vi "loadDataNodeEnd.vi"(8 "error in (no error)":errorcluster, 10 "XML Refnum in":refnum<file>, 11 "FPGADMAChannelData in":refnum<class "FPGADMAChannelData.lvclass">) -> (0 "error out":errorcluster, 2 "XML Refnum out":refnum<file>, 3 "FPGADMAChannelData out":refnum<class "FPGADMAChannelData.lvclass">)   [LabVIEW 2013, in "FPGADMAChannelData.lvclass"]
doc: "Part of the file loading process. Occurs at the end of a node being loaded. Includes checking the end of the tag which has the format </tag>."
uses:
  FPGADMAChannelData.lvclass
  xCE/xceRootNode/xceRootNode.lvclass
  XML Parser/XML Parser.lvclass
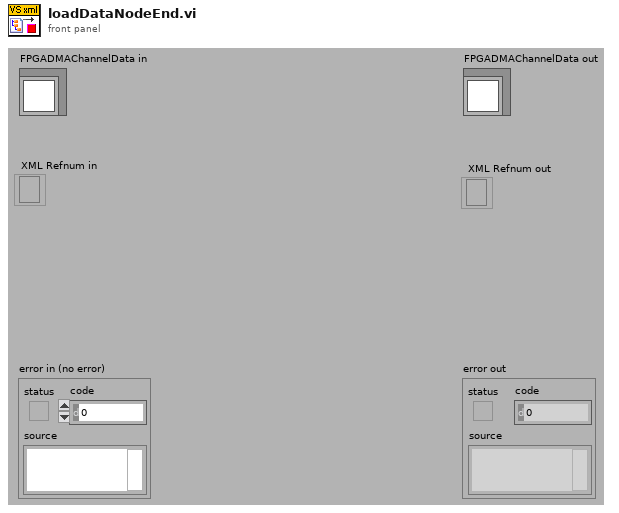
[diagram p1: front panel]
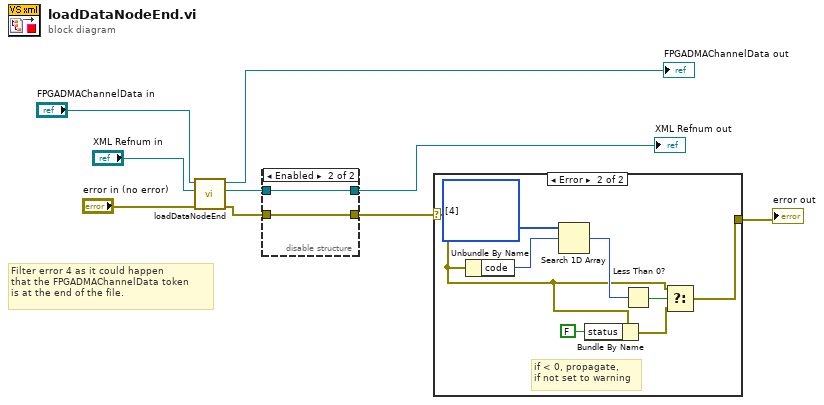
[diagram p0: block diagram]
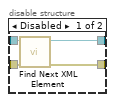
[diagram p2: hidden frame]
diagram:
  # "Filter error 4 as it could happen \nthat the FPGADMAChannelData token\nis at the end of the file."
  n1 = call-parent "loadDataNodeEnd.vi"("error in (no error)"="error in (no error)", "XML Refnum in"="XML Refnum in", "xceDataNode in"="FPGADMAChannelData in") -> ("error out"=w3:errorcluster, "XML Refnum out"=w4:refnum<file>, "xceDataNode out"=→"FPGADMAChannelData out":refnum<class "FPGADMAChannelData.lvclass">)  [unwired: 6 in]
  n2 = disable-structure shown="Enabled" {
    disable-tunnel: w4 -> [w13 w15]
    disable-tunnel: w3 -> [w12 w14]
    disable-tunnel: [w11 w15] -> w2
    disable-tunnel: [w10 w14] -> w1
    frame Disabled {
      n3 = call "Find Next XML Element.vi"("error in (no error)"=w12, "XML Fine In"=w13) -> ("error out"=w10:errorcluster, "XML Fine Out"=w11:refnum<file>)  [unwired: 7 in, 1 out]
    }
    frame Enabled {
    }
  }
  "XML Refnum out" <- w2
  n4 = case shown="Error" w1 {
    selector: w1 -> [w16 w20]
    tunnel: [w16 w17] -> w5
    frame No Error {
    }
    frame Error {
      # "if < 0, propagate,\nif not set to warning"
      n5 = Unbundle By Name(w20) -> ("code"=w23:i32)
      n6 = Search 1D Array(1D array=i32[] [4], element=w23) -> (index of element=w22:i32)  [unwired: 1 in]
      n7 = Bundle By Name(cluster=w20, "status"=FALSE) -> (w19:errorcluster)
      n8 = Less Than 0?(x=w22) -> (x < 0?=w21:bool)
      n9 = Select(t=w20, s=w21, f=w19) -> (s? t:f=w17:errorcluster)
    }
  }
  "error out" <- w5
